vi "write IMAQ keys.vi"(8 "error in (no error)":errorcluster, 11 "Point Grey Camera in":refnum<class "Point Grey Camera.lvclass">) -> (0 "error out":errorcluster, 3 "Point Grey Camera out":refnum<class "Point Grey Camera.lvclass">)   [LabVIEW 2020, in "Point Grey Camera.lvclass"]
uses:
  Point Grey Camera.lvclass
  Point Grey Camera.lvclass/Point Grey Camera.ctl
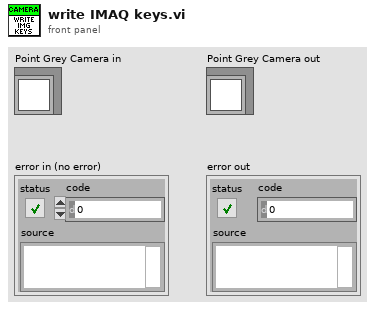
[diagram p1: front panel]
types:
  T1 = typedef "IMAQ Image.ctl" = refnum<image>
  T2 = cluster{"Value":dbl, "Min":dbl, "Max":dbl, "StepSize":dbl, "Tolerance":dbl, "valueactual":dbl}
  T3 = typedef "ROI_TypDef.ctl" = cluster{"Width":cluster{"Value":dbl, "Min":dbl, "Max":dbl, "StepSize":dbl, "Tolerance":dbl, "valueactual":dbl}, "Height":cluster{"Value":dbl, "Min":dbl, "Max":dbl, "StepSize":dbl, "Tolerance":dbl, "valueactual":dbl}, "OffsetX":cluster{"Value":dbl, "Min":dbl, "Max":dbl, "StepSize":dbl, "Tolerance":dbl, "valueactual":dbl}, "OffsetY":cluster{"Value":dbl, "Min":dbl, "Max":dbl, "StepSize":dbl, "Tolerance":dbl, "valueactual":dbl}}
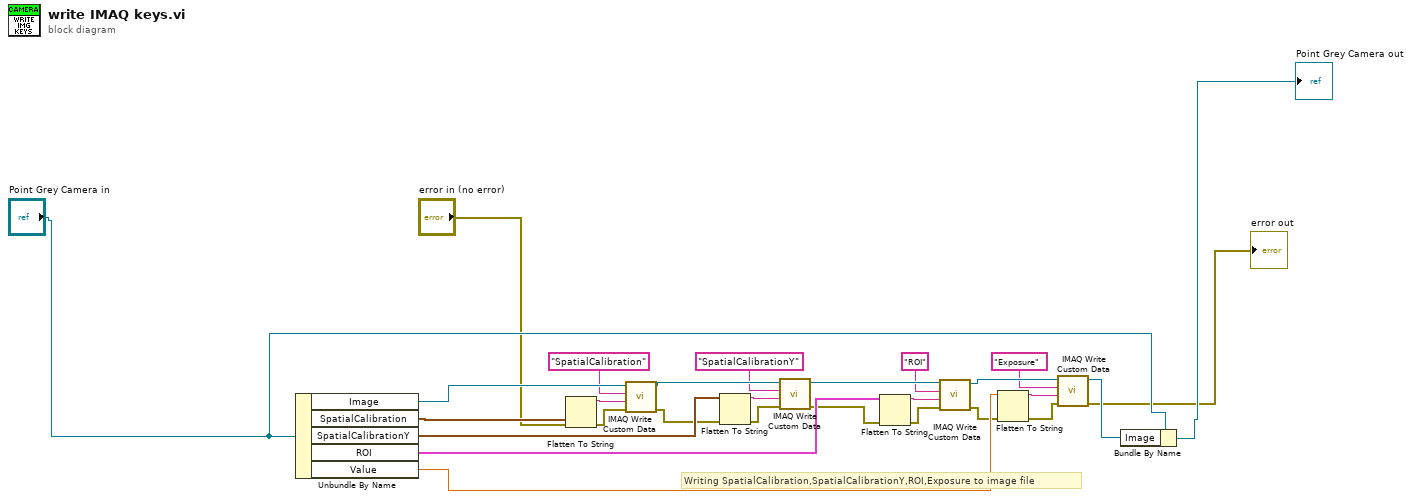
[diagram p0: block diagram]
diagram:
  # "Writing SpatialCalibration,SpatialCalibrationY,ROI,Exposure to image file"
  n1 = Unbundle By Name("Point Grey Camera in") -> ("Image"=w26:T1, "SpatialCalibration"=w22:T2, "SpatialCalibrationY"=w23:T2, "ROI"=w24:T3, "Value"=w25:dbl)
  n2 = Flatten To String(anything=w22, error in (no error)="error in (no error)") -> (data string=w2:string, error out=w9:errorcluster)  [unwired: 2 in, 1 out]
  n3 = call "IMAQ Write Custom Data"("error in (no error)"=w9, "Custom Data In"=w2, "Key"="SpatialCalibration", "Image"=w26) -> ("error out"=w21:errorcluster, "Image Out"=w18:T1)  [unwired: 6 in]
  n4 = Flatten To String(anything=w23, error in (no error)=w21) -> (data string=w16:string, error out=w15:errorcluster)  [unwired: 2 in, 1 out]
  n5 = call "IMAQ Write Custom Data"("error in (no error)"=w15, "Custom Data In"=w16, "Key"="SpatialCalibrationY", "Image"=w18) -> ("error out"=w20:errorcluster, "Image Out"=w19:T1)  [unwired: 6 in]
  n6 = Flatten To String(anything=w24, error in (no error)=w20) -> (data string=w3:string, error out=w10:errorcluster)  [unwired: 2 in, 1 out]
  n7 = call "IMAQ Write Custom Data"("error in (no error)"=w10, "Custom Data In"=w3, "Key"="ROI", "Image"=w19) -> ("error out"=w11:errorcluster, "Image Out"=w7:T1)  [unwired: 6 in]
  n8 = Flatten To String(anything=w25, error in (no error)=w11) -> (data string=w6:string, error out=w12:errorcluster)  [unwired: 2 in, 1 out]
  n9 = call "IMAQ Write Custom Data"("error in (no error)"=w12, "Custom Data In"=w6, "Key"="Exposure", "Image"=w7) -> ("error out"=→"error out":errorcluster, "Image Out"=w14:T1)  [unwired: 6 in]
  n10 = Bundle By Name(cluster="Point Grey Camera in", "Image"=w14) -> (→"Point Grey Camera out":refnum<class "Point Grey Camera.lvclass">)
